vi "SLSC Convert EDS Property to SLSC Channel Path.vi"(0 "property":T2, 1 "GUID Get Properties Page":string, 2 "GUID Set Properties Page":string, 5 "Physical Channel":string, 12 "enums":T1[](array[typedef])) -> (3 "GUID Properties Page":string, 4 "name":string, 6 "Channel out":T3, 8 "SLSC Channel Path":string="Bool.LED1.NI.GreenBool", 10 "documentation-en":string, 14 "description-en":string)   [LabVIEW 2017, in "SLSC CD System Explorer.lvlib"]
uses:
  SLSC CD API/SLSC CD System Explorer/SLSC CD System Explorer.lvlib
  <vilib>/NI Veristand/Custom Device API/Custom Device Channel.ctl
  <vilib>/NI Veristand/Custom Device API/Custom Device Channel Type.ctl
  JSON parsing/property.ctl
  JSON parsing/enum.ctl
  <vilib>/NI Veristand/Custom Device API/Custom Device API.lvlib
  SLSC CD API/SLSC CD Shared/SLSC CD Shared.lvlib
  SLSC UI API/SLSC Tree Control.lvlib
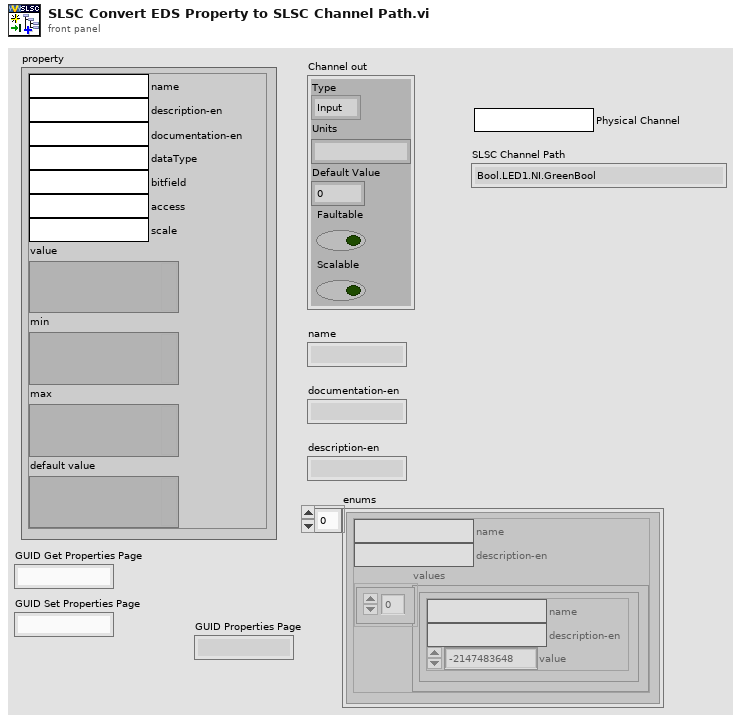
[diagram p1: front panel]
types:
  T1 = typedef "enum.ctl" = cluster{"name":string, "description-en":string, "values":cluster{"name":string, "description-en":string, "value":i32}[]}
  T2 = typedef "property.ctl" = cluster{"name":string, "description-en":string, "documentation-en":string, "dataType":string, "bitfield":string, "access":string, "scale":string, "value":variant, "min":variant, "max":variant, "default value":variant}
  T3 = typedef "Custom Device API.lvlib/Custom Device Channel.ctl" = cluster{"Type":T4, "Units":string, "Default Value":dbl, "Faultable":bool, "Scalable":bool}
  T4 = typedef "Custom Device API.lvlib/Custom Device Channel Type.ctl" = enum16{"Input", "Output"}
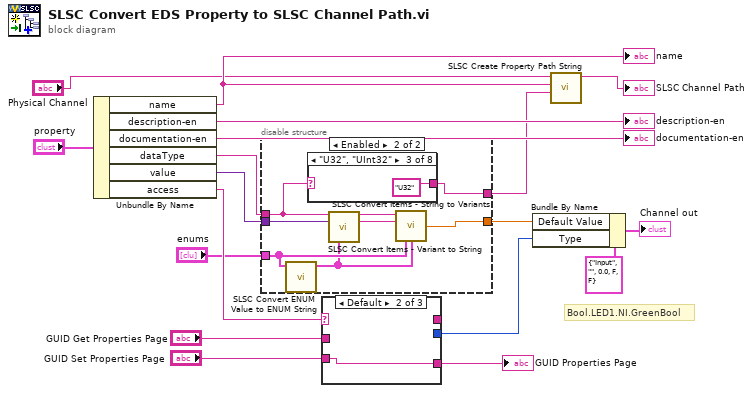
[diagram p0: block diagram]
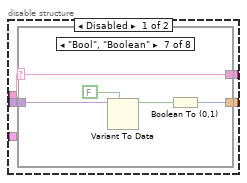
[diagram p2: hidden frame]
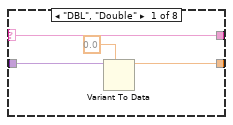
[diagram p3: hidden frame]
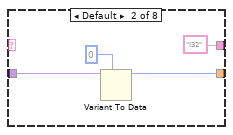
[diagram p4: hidden frame]
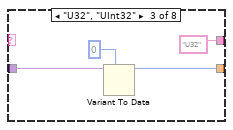
[diagram p5: hidden frame]
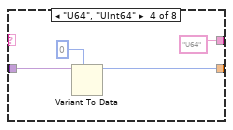
[diagram p6: hidden frame]
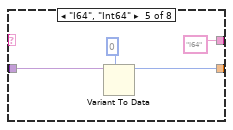
[diagram p7: hidden frame]
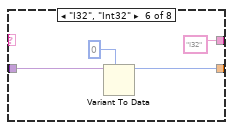
[diagram p8: hidden frame]
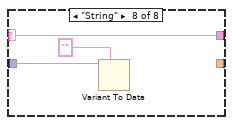
[diagram p9: hidden frame]
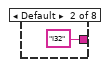
[diagram p11: hidden frame]
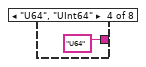
[diagram p12: hidden frame]
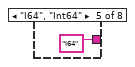
[diagram p13: hidden frame]
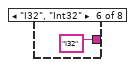
[diagram p14: hidden frame]
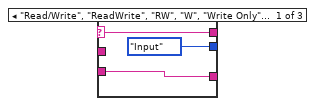
[diagram p17: hidden frame]
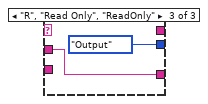
[diagram p18: hidden frame]
diagram:
  # "Bool.LED1.NI.GreenBool"
  n1 = Unbundle By Name("property") -> ("name"=w10:string, "description-en"=→"description-en":string, "documentation-en"=→"documentation-en":string, "dataType"=w13:string, "value"=w12:variant, "access"=w5:string)
  "name" <- w10
  n2 = disable-structure shown="Enabled" {
    disable-tunnel: w13 -> [w22 w56]
    disable-tunnel: w12 -> [w21 w60]
    disable-tunnel: [w20 w59] -> w11
    disable-tunnel: [w19 w55] -> w7
    disable-tunnel: "enums" -> [_ w58]
    frame Disabled {
      n3 = case shown="\"Bool\", \"Boolean\"" w22 {
        selector: w22 -> [w23 _ _ _ _ _ w47 w53]
        tunnel: w21 -> [w26 w28 w34 w38 w42 w46 w51 w54]
        tunnel: [w24 w27 w32 w36 w40 w44 w48 _] -> w20
        tunnel: [w23 "I32" "U32" "U64" "I64" "I32" w47 w53] -> w19
        frame "DBL", "Double" {
          n4 = Variant To Data(type=0.0, Variant=w26) -> (data=w24:dbl)  [unwired: 1 in, 1 out]
        }
        frame Default {
          n5 = Variant To Data(type=0, Variant=w28) -> (data=w27:i32)  [unwired: 1 in, 1 out]
        }
        frame "U32", "UInt32" {
          n6 = Variant To Data(type=u32 0, Variant=w34) -> (data=w32:u32)  [unwired: 1 in, 1 out]
        }
        frame "U64", "UInt64" {
          n7 = Variant To Data(type=u64 0, Variant=w38) -> (data=w36:u64)  [unwired: 1 in, 1 out]
        }
        frame "I64", "Int64" {
          n8 = Variant To Data(type=i64 0, Variant=w42) -> (data=w40:i64)  [unwired: 1 in, 1 out]
        }
        frame "I32", "Int32" {
          n9 = Variant To Data(type=0, Variant=w46) -> (data=w44:i32)  [unwired: 1 in, 1 out]
        }
        frame "Bool", "Boolean" {
          n10 = Variant To Data(type=FALSE, Variant=w51) -> (data=w49:bool)  [unwired: 1 in, 1 out]
          n11 = Boolean To (0,1)(Boolean=w49) -> (0, 1=w48:i16)
        }
        frame "String" {
          n12 = Variant To Data(type="", Variant=w54) -> ()  [unwired: 1 in, 2 out]
        }
      }
    }
    frame Enabled {
      n13 = call "SLSC Convert ENUM Value to ENUM String.vi"("enums"=w58) -> ("string enums"=w57:cluster{"name":string, "string enums":string}[])  [unwired: 10 in]
      n14 = case shown="\"U32\", \"UInt32\"" w56 {
        selector: w56 -> [w63 _ _ _ _ _ w69 w70]
        tunnel: [w63 "I32" "U32" "U64" "I64" "I32" w69 w70] -> w55
        frame "DBL", "Double" {
        }
        frame Default {
        }
        frame "U32", "UInt32" {
        }
        frame "U64", "UInt64" {
        }
        frame "I64", "Int64" {
        }
        frame "I32", "Int32" {
        }
        frame "Bool", "Boolean" {
        }
        frame "String" {
        }
      }
      n15 = call "SLSC Convert Items - Variant to String.vi"("dataType"=w56, "value"=w60, "Enum string"=w57) -> ("Output data type"=w62:string, "string data value"=w61:string)  [unwired: 6 in, 5 out]
      n16 = call "SLSC Convert Items - String to Variants.vi"("Datatype"=w62, "Value"=w61, "enums"=w58, "string enums"=w57) -> ("Value (DBL)"=w59:dbl)  [unwired: 8 in, 3 out]
    }
  }
  n17 = case shown="Default" w5 {
    selector: w5 -> [w72 _ _]
    tunnel: [Custom_Device_Channel_Type."Input" ("Type") _ Custom_Device_Channel_Type."Output" ("Type")] -> w6
    tunnel: [w72 _ _] -> _
    tunnel: [w71 w74 w75] -> w4
    tunnel: "GUID Set Properties Page" -> [w71 w74 _]
    tunnel: "GUID Get Properties Page" -> [_ _ w75]
    frame "Read/Write", "ReadWrite", "RW", "W", "Write Only", "WriteOnly" {
    }
    frame Default {
    }
    frame "R", "Read Only", "ReadOnly" {
    }
  }
  "GUID Properties Page" <- w4
  n18 = Bundle By Name(cluster=T3 {"Type"=enum."Input", "Units"="", "Default Value"=0.0, "Faultable"=FALSE, "Scalable"=FALSE} ("Channel out"), "Default Value"=w11, "Type"=w6) -> (→"Channel out":T3)
  n19 = call "SLSC Create Property Path String.vi"("Datatype"=w7, "Property"=w10, "Physical Channel"="Physical Channel") -> ("SLSC Path String"=→"SLSC Channel Path":string)  [unwired: 8 in]
